vi "rad_Load Config.vi"(8 "error in (no error":errorcluster, 11 "State in":T1 {"Targets Information"."Primary NIC"."IP Address Request Mode" items=["Static"=1, "DHCP/Link-Local"=2, "Link-Local Only"=4, "DHCP Only"=8]}) -> (0 "error out":errorcluster, 3 "State out":T1 {"Targets Information"."Primary NIC"."IP Address Request Mode" items=["Static"=1, "DHCP/Link-Local"=2, "Link-Local Only"=4, "DHCP Only"=8]})   [LabVIEW 2020]
uses:
  TypeDefs/rad_State Data.ctl
  Targets/TypeDefs/rad_Targets Settings.ctl
  Targets/TypeDefs/rad_Target Information.ctl
  Targets/TypeDefs/rad_Target Network Settings.ctl
  App Images/TypeDefs/rad_App Images Settings.ctl
  App Images/TypeDefs/rad_AppImage Information.ctl
  App Images/TypeDefs/rad_Application Image Properties.ctl
  App Images/TypeDefs/rad_FPGA Properties.ctl
  App Images/TypeDefs/rad_FPGA Flash Properties.ctl
  <vilib>/Utility/config.llb/Read Key (Path).vi
  <vilib>/Utility/config.llb/Read Key (Boolean).vi
  <vilib>/Utility/config.llb/Read Key (String).vi
  <vilib>/Utility/config.llb/Read Key (I32).vi
  <vilib>/Utility/config.llb/NI_LVConfig.lvlib
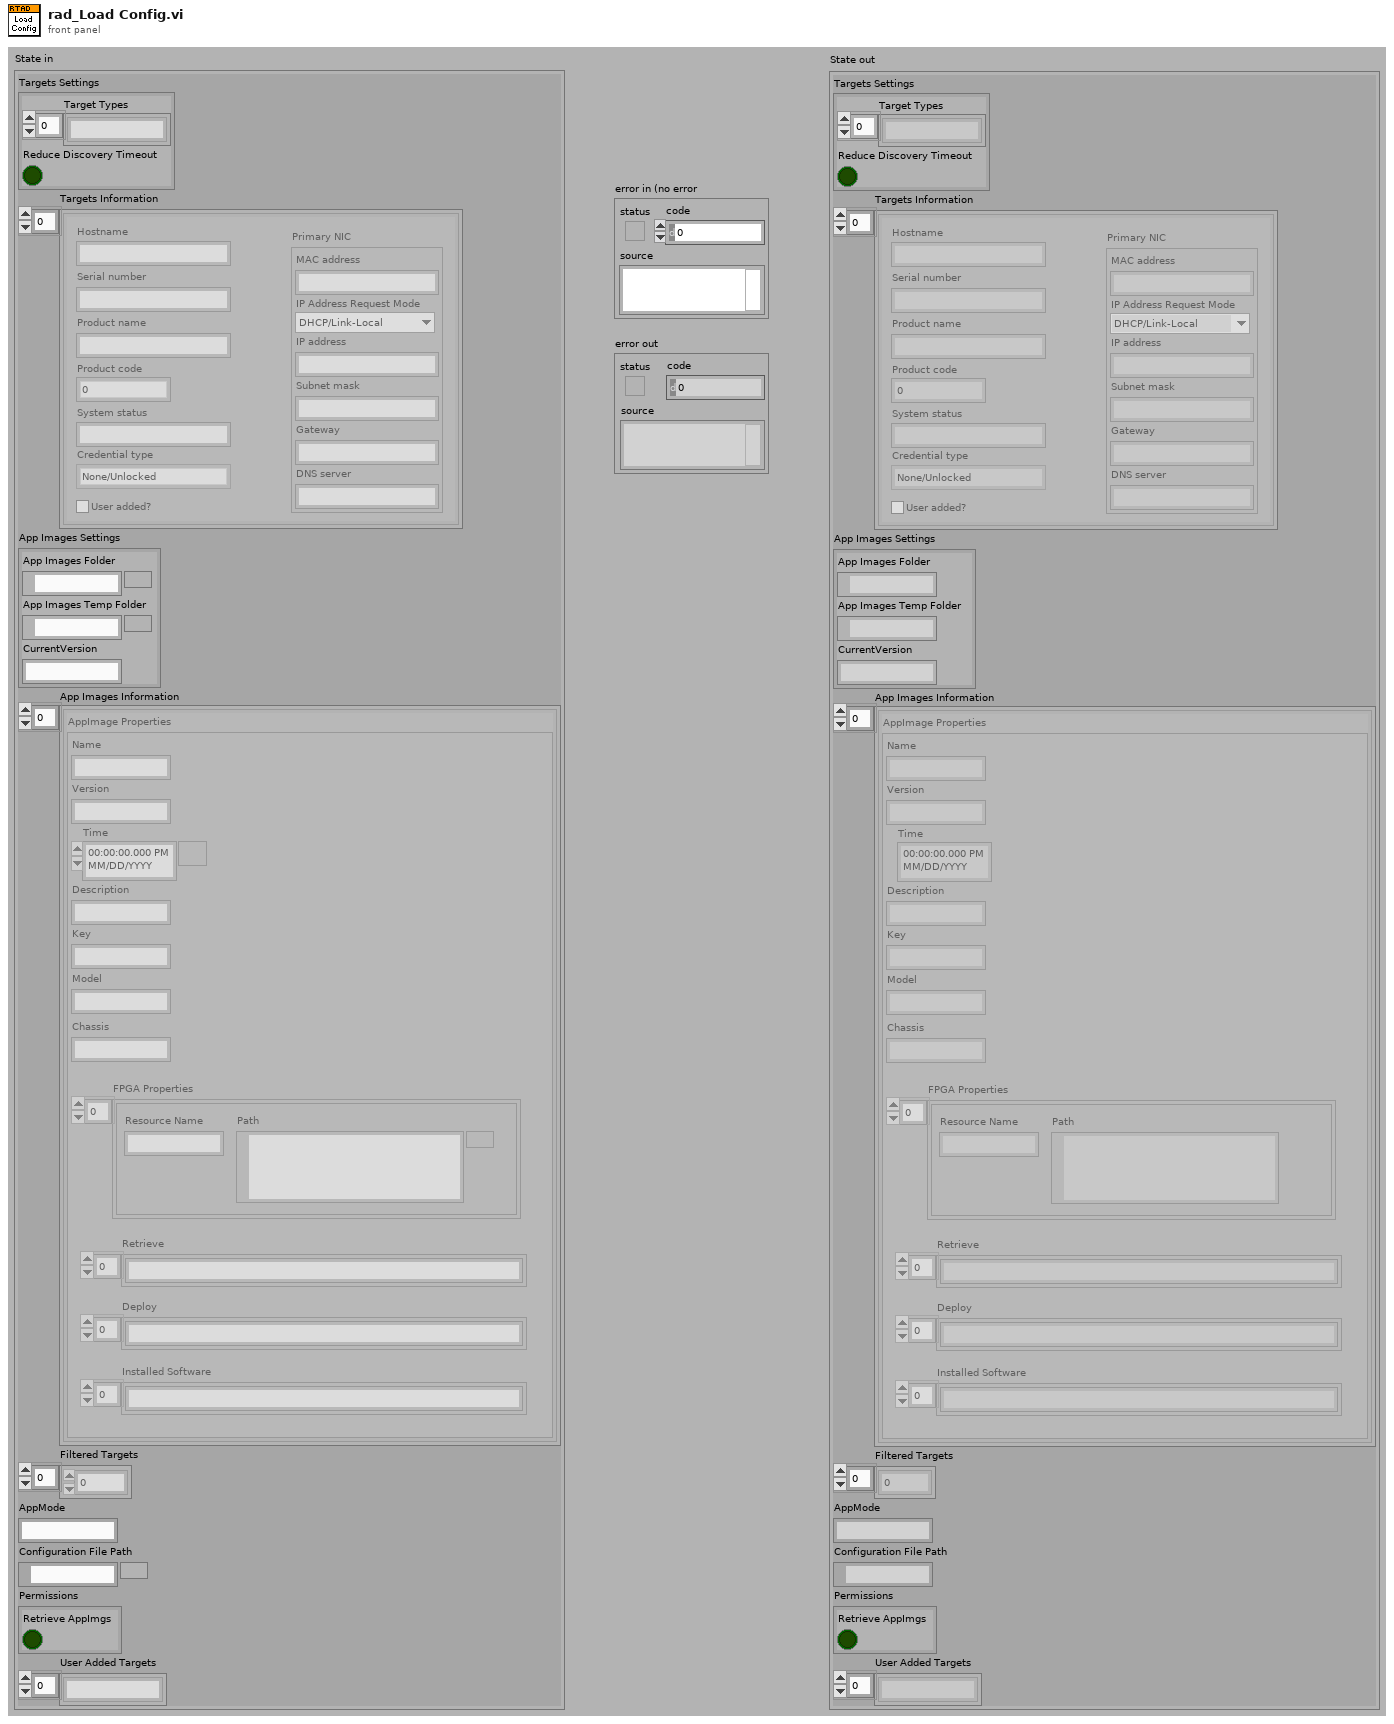
[diagram p1: front panel]
types:
  T1 = typedef "rad_State Data.ctl" = cluster{"Targets Settings":T2, "Targets Information":T3[], "App Images Settings":T5, "App Images Information":T6[], "Filtered Targets":i32[], "AppMode":string, "Configuration File Path":path, "Permissions":cluster{"Retrieve AppImgs":bool}, "User Added Targets":string[]}
  T2 = typedef "rad_Targets Settings.ctl" = cluster{"Target Types":string[], "Reduce Discovery Timeout":bool}
  T3 = typedef "rad_Target Information.ctl" = cluster{"Hostname":string, "Serial number":string, "Product name":string, "Product code":i32, "System status":string, "Credential type":enum16{"None/Unlocked", "FTP Password", "NIAuth Credentials"}, "User added?":bool, "Primary NIC":T4}
  T4 = typedef "rad_Target Network Settings.ctl" = cluster{"MAC address":string, "IP Address Request Mode":i32, "IP address":string, "Subnet mask":string, "Gateway":string, "DNS server":string}
  T5 = typedef "rad_App Images Settings.ctl" = cluster{"App Images Folder":path, "App Images Temp Folder":path, "CurrentVersion":string}
  T6 = typedef "rad_AppImage Information.ctl" = cluster{"AppImage Properties":T7, "AppImage Path":path}
  T7 = typedef "rad_Application Image Properties.ctl" = cluster{"Name":string, "Version":string, "Time":timestamp, "Description":string, "Key":string, "Chassis":string, "FPGA Properties":T8, "Model":string, "Retrieve":string[], "Deploy":string[], "Installed Software":string[]}
  T8 = typedef "rad_FPGA Properties.ctl" = T9[]
  T9 = typedef "rad_FPGA Flash Properties.ctl" = cluster{"Resource Name":string, "Path":path}
  T10 = typedef "NI_LVConfig.lvlib/Config Data RefNum.ctl" = refnum<k1>
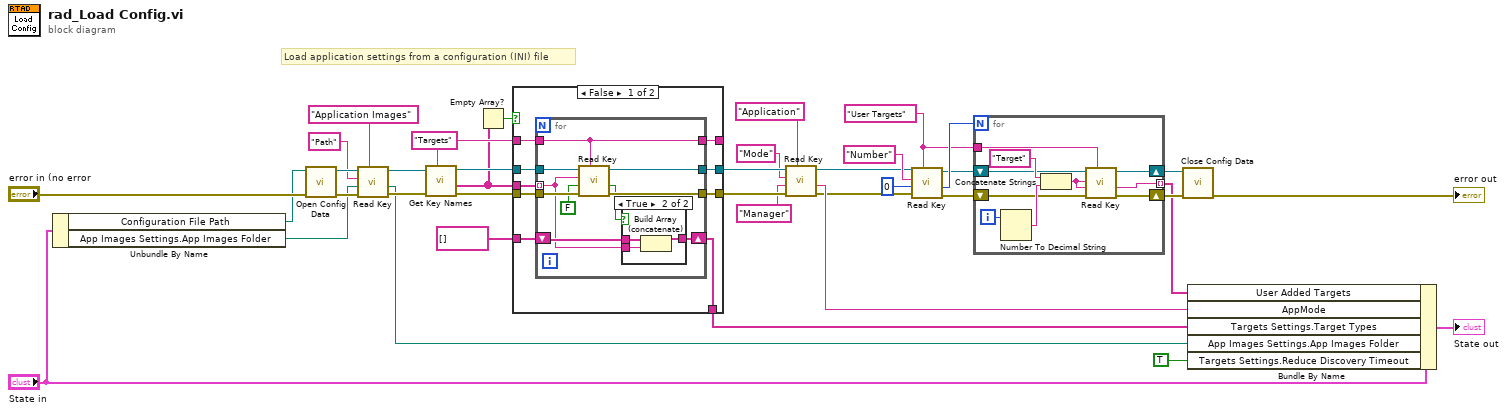
[diagram p0: block diagram]
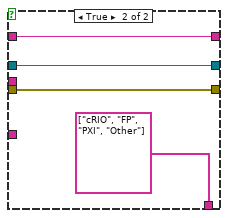
[diagram p3: hidden frame]
diagram:
  w12 = "User Targets" ("section")
  w31 = "Targets" ("section")
  # "Load application settings from a configuration (INI) file"
  n1 = Unbundle By Name("State in") -> ("Configuration File Path"=w2:path, "App Images Settings.App Images Folder"=w17:path)
  n2 = call <vilib>:"Open Config Data.vi"("error in (no error)"="error in (no error", "configuration file path"=w2) -> ("error out"=w38:errorcluster, "refnum"=w37:T10)  [unwired: 7 in, 1 out]
  n3 = call-poly <vilib>:"Read Key.vi"("section"="Application Images", "error in (no error)"=w38, "default value"=w17, "key"="Path", "refnum"=w37) -> ("error out"=w33:errorcluster, "value"=w6:path, "refnum out"=w34:T10)  [unwired: 4 out]
  n4 = call <vilib>:"Get Key Names.vi"("section"=w31, "error in (no error)"=w33, "refnum"=w34) -> ("error out"=w32:errorcluster, "key names"=w27:string[], "refnum out"=w28:T10)  [unwired: 6 out]
  n5 = Empty Array?(array=w27) -> (empty?=w26:bool)
  n6 = case shown="False" w26 {
    tunnel: w32 -> [w47 w63]
    tunnel: w27 -> [w46 _]
    tunnel: w31 -> [w45 w65]
    tunnel: w28 -> [w44 w64]
    tunnel: [w41 w65] -> _
    tunnel: [w43 w64] -> w21
    tunnel: [w42 w63] -> w20
    tunnel: string[] [] ("Targets") -> [w40 _]
    tunnel: [w39 string[] ["cRIO", "FP", "PXI", "Other"] ("Targets")] -> w23
    frame False {
      n7 = for {
        tunnel: w47 -> [w57]
        tunnel: w44 -> [w55]
        tunnel: w46 -> [w48] mode=indexing
        tunnel: w45 -> [w56]
        tunnel: [w56] -> w41
        tunnel: [w54] -> w42
        tunnel: [w53] -> w43
        shift-right: [w49] -> w39
        shift-left: w40 -> [w50]
        n8 = call-poly <vilib>:"Read Key.vi"("section"=w56, "error in (no error)"=w57, "default value"=FALSE, "key"=w48, "refnum"=w55) -> ("error out"=w54:errorcluster, "value"=w51:bool, "refnum out"=w53:T10)  [unwired: 4 out]
        n9 = case shown="True" w51 {
          tunnel: w50 -> [w58 w61]
          tunnel: [w58 w60] -> w49
          tunnel: w48 -> [_ w59]
          frame False {
          }
          frame True {
            n10 = Build Array (concatenate)(w61, w59) -> (w60:string[])
          }
        }
      }
    }
    frame True {
    }
  }
  n11 = call-poly <vilib>:"Read Key.vi"("section"="Application", "error in (no error)"=w20, "default value"="Manager", "key"="Mode", "refnum"=w21) -> ("error out"=w4:errorcluster, "value"=w18:string, "refnum out"=w3:T10)  [unwired: 1 in, 3 out]
  n12 = call-poly <vilib>:"Read Key.vi"("section"=w12, "error in (no error)"=w4, "default value"=0 ("size(s)"), "key"="Number", "refnum"=w3) -> ("error out"=w11:errorcluster, "value"=w14:i32, "refnum out"=w13:T10)  [unwired: 4 out]
  n13 = for {
    N: w14 -> [_]
    tunnel: w12 -> [w69]
    shift-right: [w72] -> w9
    shift-left: w11 -> [w71]
    tunnel: [w66] -> w8 mode=indexing
    shift-right: [w67] -> w10
    shift-left: w13 -> [w68]
    i -> [w74]
    n14 = Number To Decimal String(number=w74) -> (decimal integer string=w75:string)  [unwired: 1 in]
    n15 = Concatenate Strings("Target" ("key"), w75) -> (w70:string)
    n16 = call-poly <vilib>:"Read Key.vi"("section"=w69, "error in (no error)"=w71, "default value"=w70, "key"=w70, "refnum"=w68) -> ("error out"=w72:errorcluster, "value"=w66:string, "refnum out"=w67:T10)  [unwired: 1 in, 3 out]
  }
  n17 = call <vilib>:"Close Config Data.vi"("error in (no error)"=w9, "refnum"=w10) -> ("error out"=→"error out":errorcluster)  [unwired: 1 in, 8 out]
  n18 = Bundle By Name(cluster="State in", "User Added Targets"=w8, "AppMode"=w18, "Targets Settings.Target Types"=w23, "App Images Settings.App Images Folder"=w6, "Targets Settings.Reduce Discovery Timeout"=TRUE) -> (→"State out":T1)
